vi "NI PXI-4110 Programmable Power Supply Ch Page.vi"(8 "error in (no error)":errorcluster, 11 "Node Ptr":T3 format="%.0x") -> (0 "error out":errorcluster)   [LabVIEW 2015, in "NI PXI-4110 Programmable Power Supply Custom Device.lvlib"]
uses:
  NI PXI-4110 Programmable Power Supply Custom Device.lvlib
  <vilib>/NI Veristand/Custom Device API/Custom Device Item Ref.ctl
  <instrlib>/niDCPower/nidcpower.llb/niDCPower Sense.ctl
  4110_Channel #.ctl
  4110_Global.vi
  <vilib>/NI Veristand/Custom Device API/Get Item Property (U16).vi
  <vilib>/NI Veristand/Custom Device API/Get Item Property (Double).vi
  <vilib>/NI Veristand/Custom Device API/Get Item Property (I32).vi
  <vilib>/NI Veristand/Custom Device API/Set Item Property (I32).vi
  <vilib>/NI Veristand/Custom Device API/Set Item Property (U16).vi
  <vilib>/NI Veristand/Custom Device API/Set Item Property (Double).vi
  <vilib>/NI VeriStand/Custom Device API/Custom Device API.lvlib
panel:
  in  "Channel #":T1
  in  "Voltage Limit":dbl caption="Range (0-6V)" format="%.4f"
  in  "Initial Current Value":dbl caption="Range (0.01 -1A)" format="%.4f"
  in  "Current Limit":dbl caption="Range (0.01-1A)" format="%.4f"
  in  "sense":T2=1008 caption="Sense" items=["Local"=1008, "Remote"=1009]
  in  "IO Type":enum16{"Voltage Output", "Current Output"}(ring)
  in  "Initial Voltage Value":dbl caption="Range (0-6V)" format="%_4f"
  in  "Name":string
  in  "Header":cluster{"Section Name":string}={"Section Name"="PXI-4110  Settings"}
  in  "Description":string
  in  "Delete":bool
  # "Voltage  IO Settings"
  # "Current IO Settings"
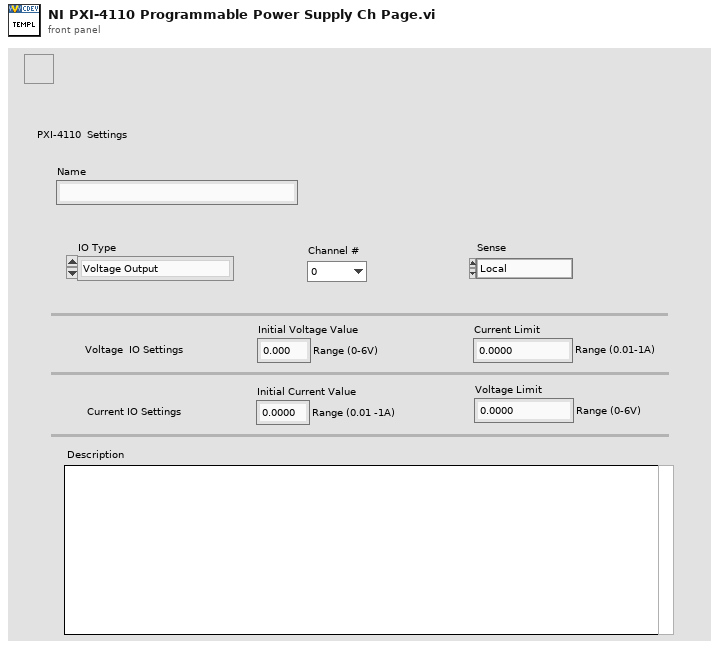
[diagram p1: front panel]
types:
  T1 = typedef "NI PXI-4110 Programmable Power Supply Custom Device.lvlib/4110_Channel #.ctl" = enum16{"0", "1", "2"}
  T2 = typedef "niDCPower Sense.ctl" = i32
  T3 = typedef "Custom Device API.lvlib/Custom Device Item Ref.ctl" = u64
  T4 = enum8{"Enabled", "Disabled", "Disabled and Grayed Out"}
  T5 = typedef "Custom Device API.lvlib/Custom Device Item Info.ctl" = cluster{"Name":string, "Is Channel":bool, "GUID":string, "Is Waveform":bool}
  T6 = cluster{"V_min":dbl, "V_max":dbl, "I_min":dbl, "I_max":dbl}
  T7 = typedef "Custom Device API.lvlib/Custom Device Commands.ctl" = enum16{"Default", "Item renamed", "Shutdown", "Dynamic button pressed"}
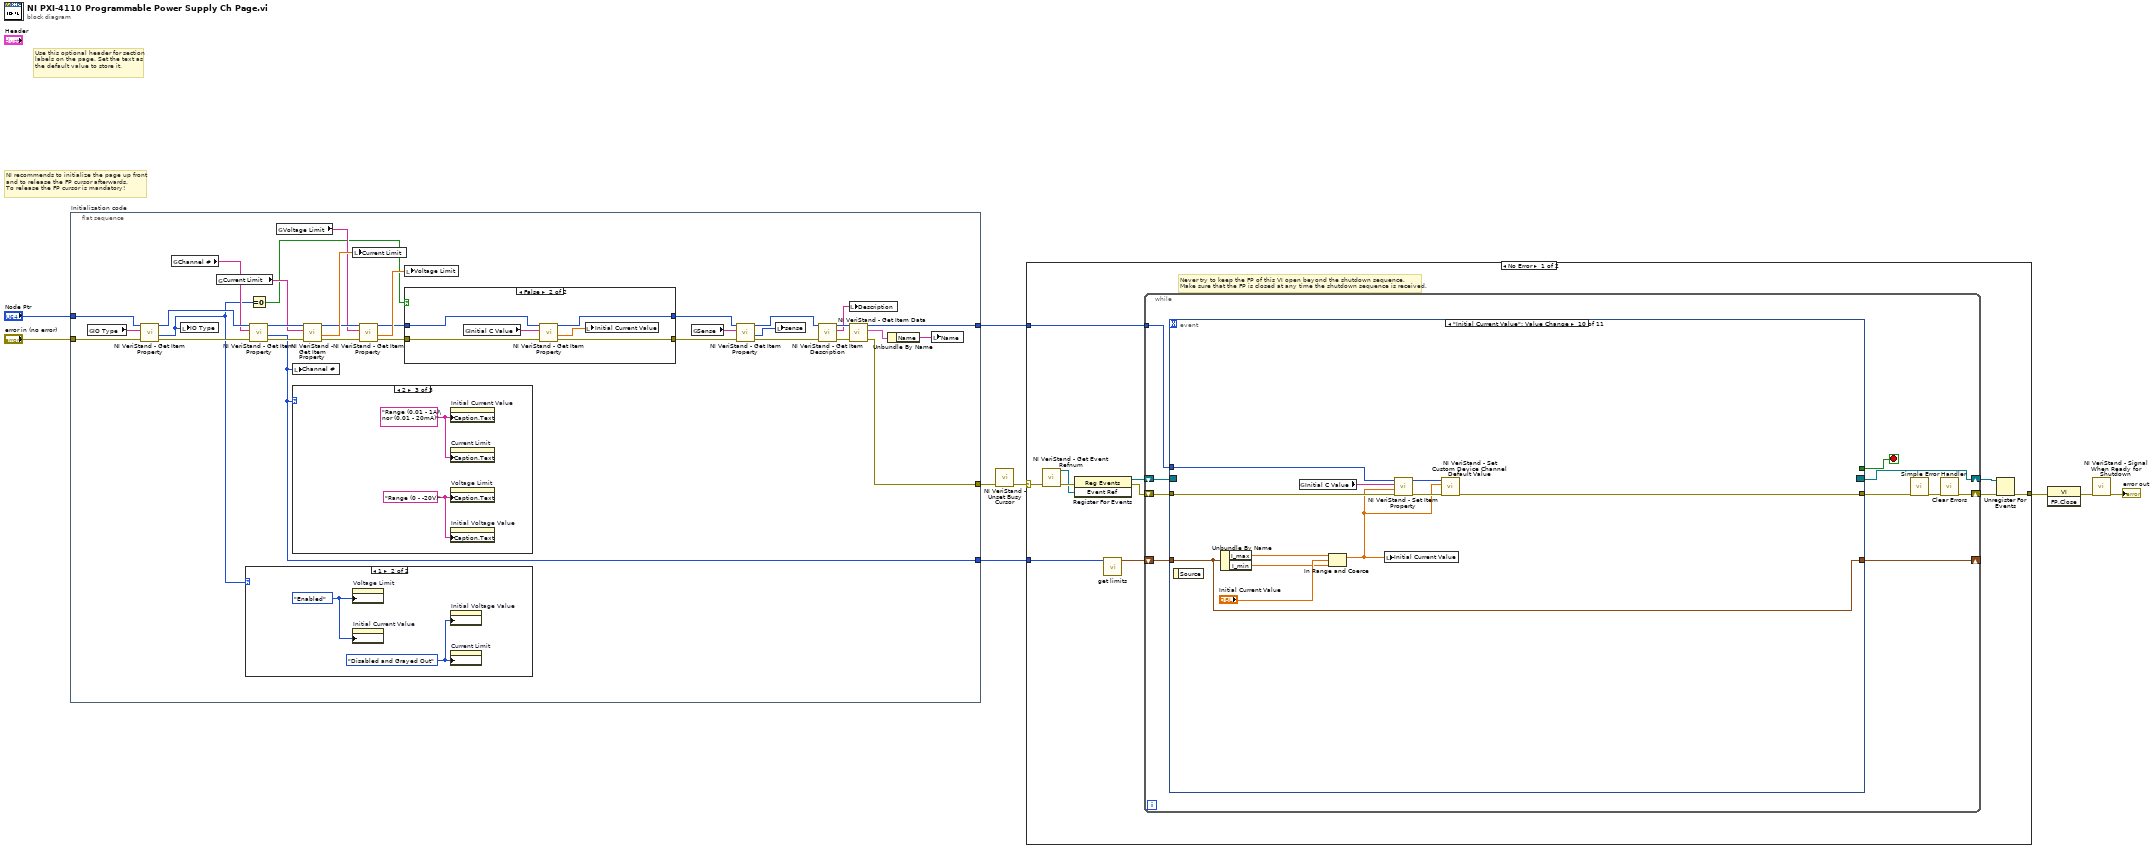
[diagram p0: block diagram]
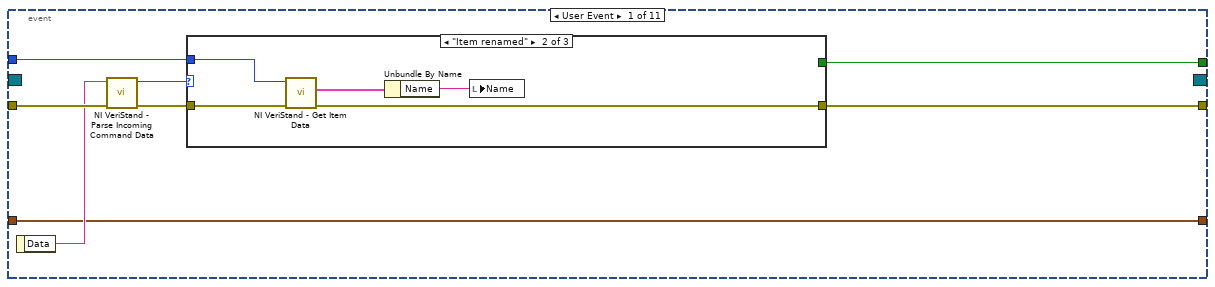
[diagram p2: hidden frame]
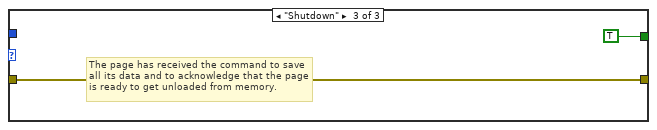
[diagram p4: hidden frame]
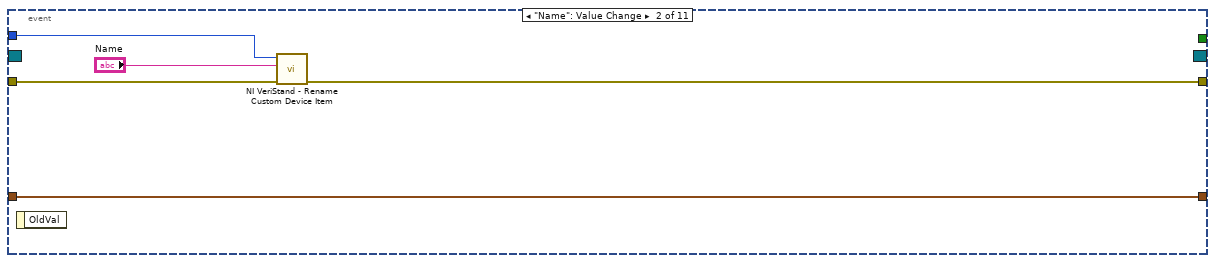
[diagram p5: hidden frame]
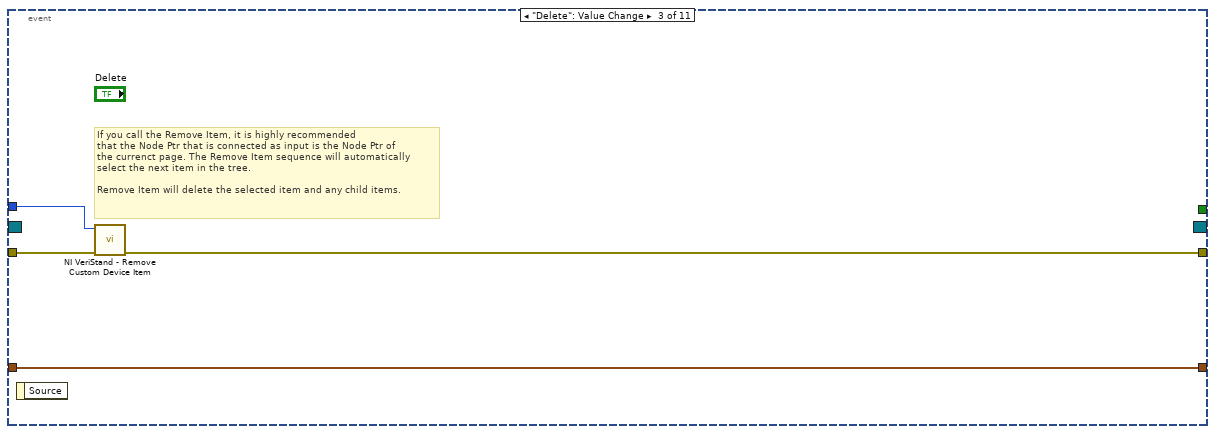
[diagram p6: hidden frame]
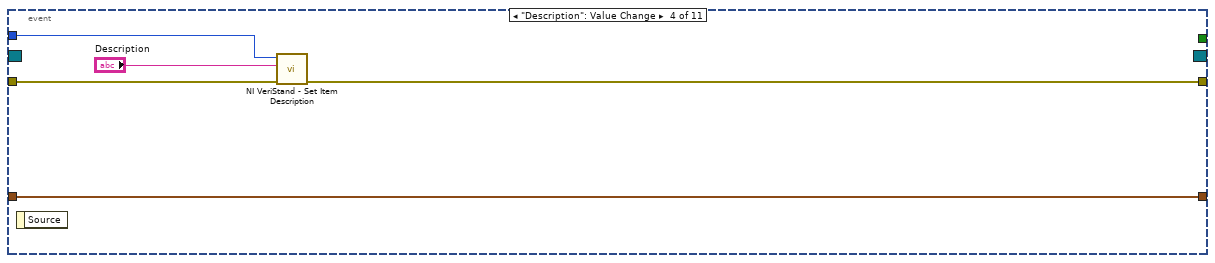
[diagram p7: hidden frame]
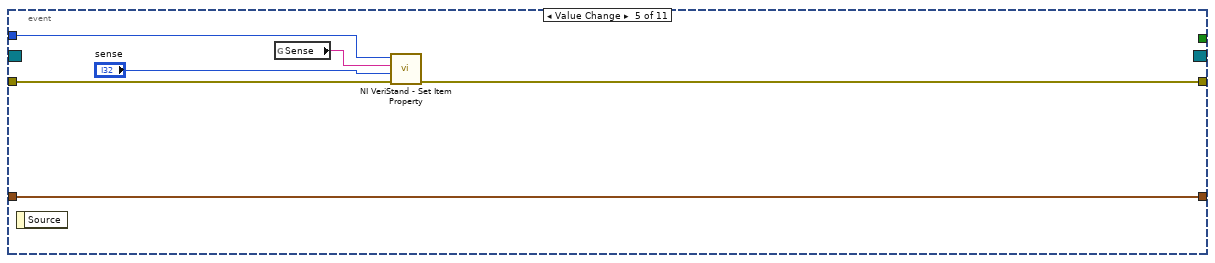
[diagram p8: hidden frame]
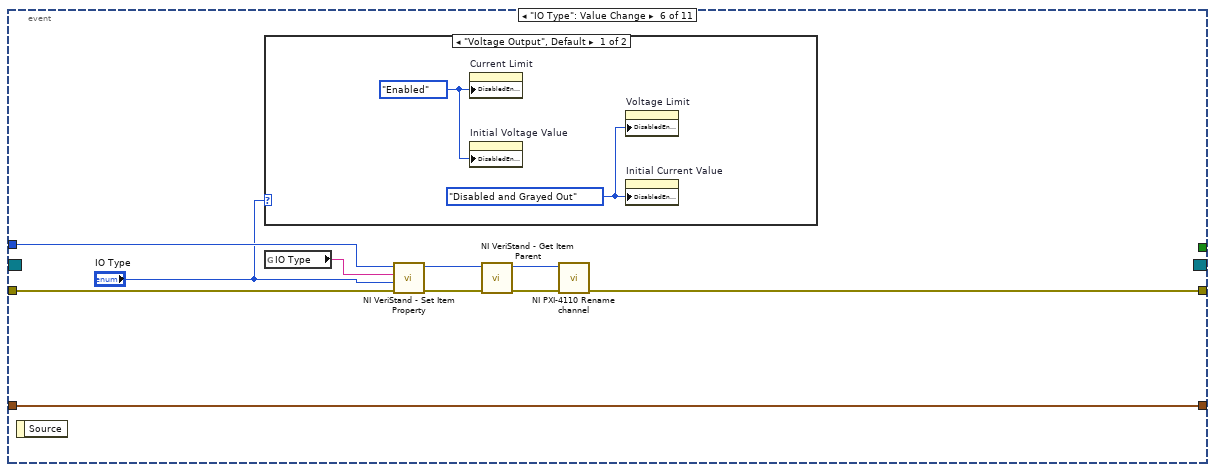
[diagram p9: hidden frame]
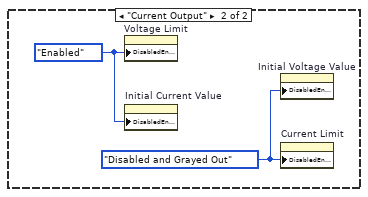
[diagram p10: hidden frame]
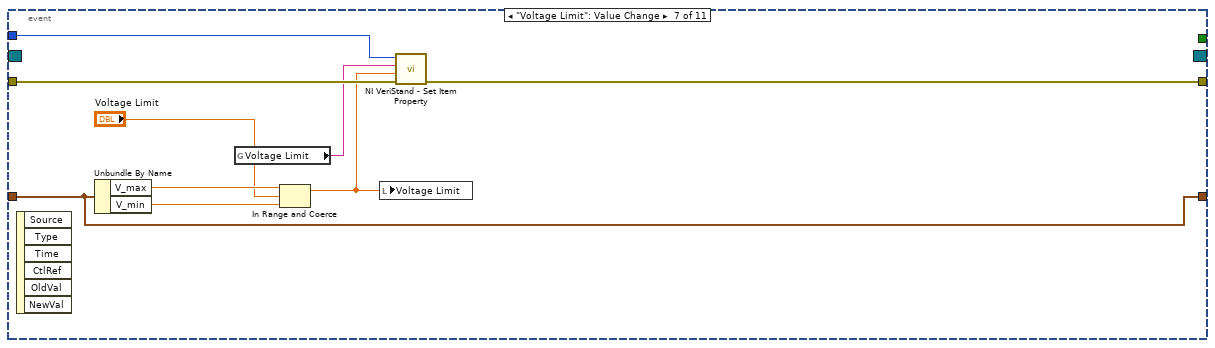
[diagram p11: hidden frame]
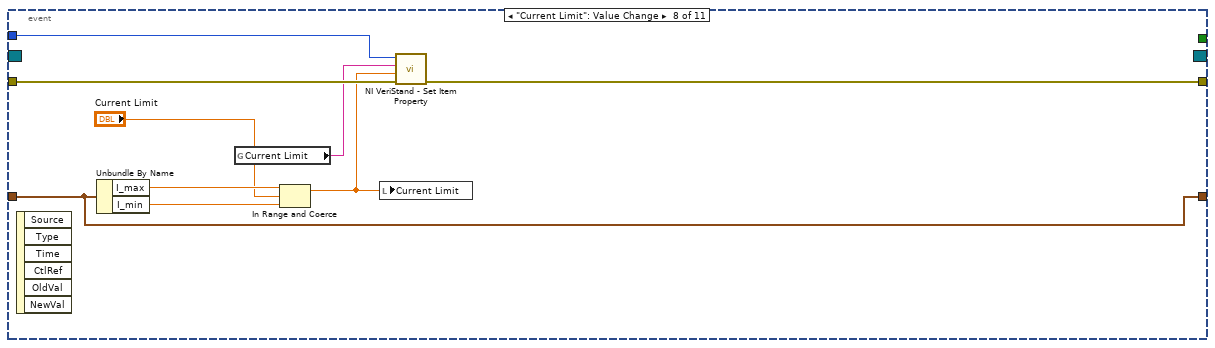
[diagram p12: hidden frame]
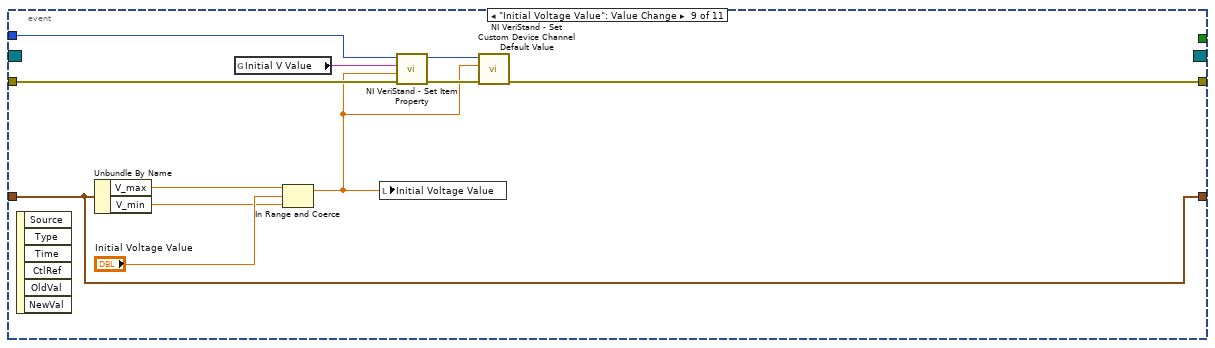
[diagram p13: hidden frame]
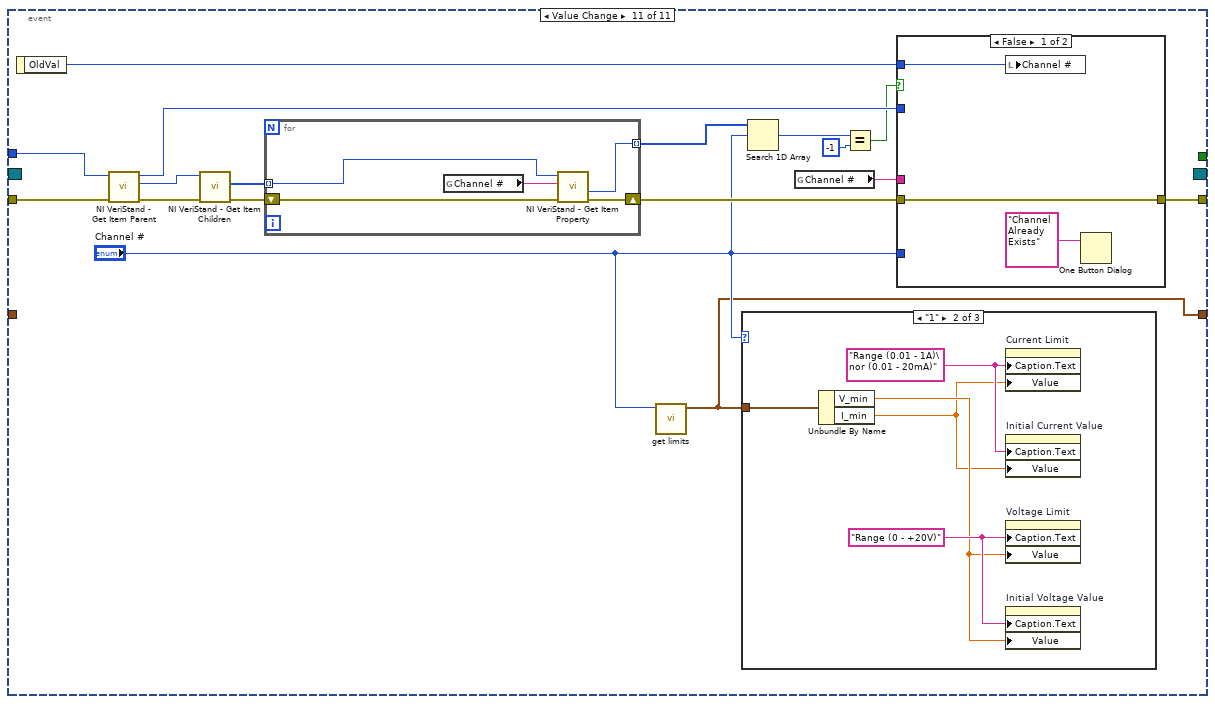
[diagram p14: hidden frame]
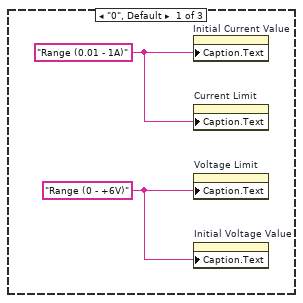
[diagram p15: hidden frame]
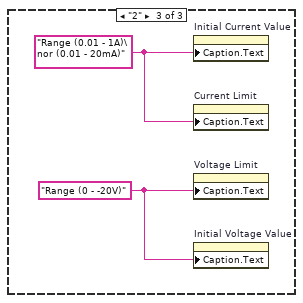
[diagram p16: hidden frame]
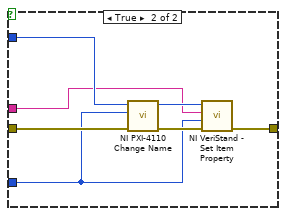
[diagram p17: hidden frame]
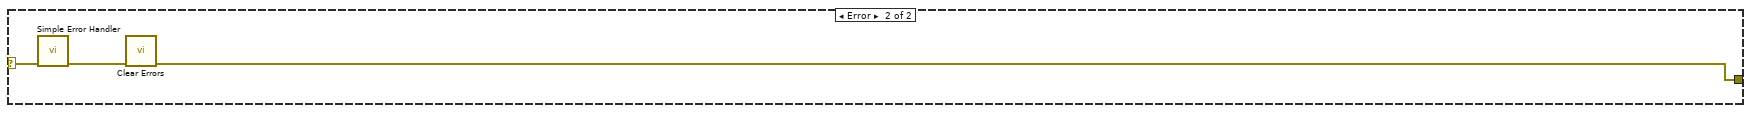
[diagram p18: hidden frame]
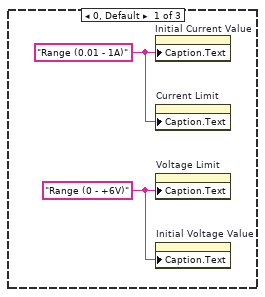
[diagram p19: hidden frame]
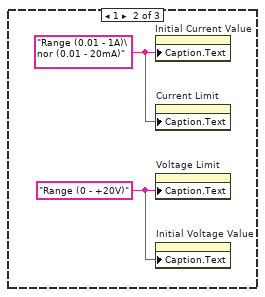
[diagram p20: hidden frame]
diagram:
  # "Use this optional header for section labels on the page. Set the text as the default value to store it."
  # "NI recommends to initialize the page up front\nand to release the FP cursor afterwards.\nTo release the FP cursor is mandatory!"
  n1 = flat-sequence "Initialization code" {
    tunnel: "error in (no error)" -> [w34]
    tunnel: "Node Ptr" -> [w33]
    tunnel: [w36] -> w5
    tunnel: [w41] -> w3
    tunnel: [w10] -> w1
    frame #0 {
      n2 = global read "4110_Global.vi" "IO Type"() -> (w32:string)
      n3 = call-poly <vilib>:"NI VeriStand - Get Item Property.vi"("error in (no error)"=w34, "Property Name"=w32, "Item Ref in"=w33) -> ("error out"=w31:errorcluster, "Value"=w12:u16, "Item Ref out"=w30:T3)  [unwired: 5 in, 1 out]
      n4 = global read "4110_Global.vi" "Channel #"() -> (w29:string)
      n5 = local write "IO Type"(w12) -> ()
      n6 = global read "4110_Global.vi" "Current Limit"() -> (w26:string)
      n7 = case shown="1" w12 {
        frame 0, Default {
          w60 = T4."Enabled" ("Disabled")
          w61 = T4."Disabled and Grayed Out" ("Disabled")
          n8 = property on="Current Limit" class="DigNum (strict)"("DisabledEnum"=w60) -> ()  [unwired: 2 in, 2 out]
          n9 = property on="Initial Voltage Value" class="DigNum (strict)"("DisabledEnum"=w60) -> ()  [unwired: 2 in, 2 out]
          n10 = property on="Voltage Limit" class="DigNum (strict)"("DisabledEnum"=w61) -> ()  [unwired: 2 in, 2 out]
          n11 = property on="Initial Current Value" class="DigNum (strict)"("DisabledEnum"=w61) -> ()  [unwired: 2 in, 2 out]
        }
        frame 1 {
          w62 = T4."Enabled" ("Disabled")
          w63 = T4."Disabled and Grayed Out" ("Disabled")
          n12 = property on="Voltage Limit" class="DigNum (strict)"("DisabledEnum"=w62) -> ()  [unwired: 2 in, 2 out]
          n13 = property on="Initial Current Value" class="DigNum (strict)"("DisabledEnum"=w62) -> ()  [unwired: 2 in, 2 out]
          n14 = property on="Initial Voltage Value" class="DigNum (strict)"("DisabledEnum"=w63) -> ()  [unwired: 2 in, 2 out]
          n15 = property on="Current Limit" class="DigNum (strict)"("DisabledEnum"=w63) -> ()  [unwired: 2 in, 2 out]
        }
      }
      n16 = Equal To 0?(x=w12) -> (x = 0?=w11:bool)
      n17 = call-poly <vilib>:"NI VeriStand - Get Item Property.vi"("error in (no error)"=w31, "Property Name"=w29, "Item Ref in"=w30) -> ("error out"=w27:errorcluster, "Value"=w10:u16, "Item Ref out"=w28:T3)  [unwired: 5 in, 1 out]
      n18 = global read "4110_Global.vi" "Voltage Limit"() -> (w22:string)
      n19 = local write "Channel #"(w10) -> ()
      n20 = case shown="2" w10 {
        frame 0, Default {
          w42 = "Range (0 - +6V)" ("Caption.Text")
          w43 = "Range (0.01 - 1A)" ("Caption.Text")
          n21 = property on="Initial Current Value" class="DigNum (strict)"("Caption.Text"=w43) -> ()  [unwired: 2 in, 2 out]
          n22 = property on="Current Limit" class="DigNum (strict)"("Caption.Text"=w43) -> ()  [unwired: 2 in, 2 out]
          n23 = property on="Voltage Limit" class="DigNum (strict)"("Caption.Text"=w42) -> ()  [unwired: 2 in, 2 out]
          n24 = property on="Initial Voltage Value" class="DigNum (strict)"("Caption.Text"=w42) -> ()  [unwired: 2 in, 2 out]
        }
        frame 1 {
          w44 = "Range (0 - +20V)" ("Caption.Text")
          w45 = "Range (0.01 - 1A)\nor (0.01 - 20mA)" ("Caption.Text")
          n25 = property on="Initial Current Value" class="DigNum (strict)"("Caption.Text"=w45) -> ()  [unwired: 2 in, 2 out]
          n26 = property on="Current Limit" class="DigNum (strict)"("Caption.Text"=w45) -> ()  [unwired: 2 in, 2 out]
          n27 = property on="Voltage Limit" class="DigNum (strict)"("Caption.Text"=w44) -> ()  [unwired: 2 in, 2 out]
          n28 = property on="Initial Voltage Value" class="DigNum (strict)"("Caption.Text"=w44) -> ()  [unwired: 2 in, 2 out]
        }
        frame 2 {
          w46 = "Range (0 - -20V)" ("Caption.Text")
          w47 = "Range (0.01 - 1A)\nor (0.01 - 20mA)" ("Caption.Text")
          n29 = property on="Initial Current Value" class="DigNum (strict)"("Caption.Text"=w47) -> ()  [unwired: 2 in, 2 out]
          n30 = property on="Current Limit" class="DigNum (strict)"("Caption.Text"=w47) -> ()  [unwired: 2 in, 2 out]
          n31 = property on="Voltage Limit" class="DigNum (strict)"("Caption.Text"=w46) -> ()  [unwired: 2 in, 2 out]
          n32 = property on="Initial Voltage Value" class="DigNum (strict)"("Caption.Text"=w46) -> ()  [unwired: 2 in, 2 out]
        }
      }
      n33 = call-poly <vilib>:"NI VeriStand - Get Item Property.vi"("error in (no error)"=w27, "Property Name"=w26, "Item Ref in"=w28) -> ("error out"=w24:errorcluster, "Value"=w25:dbl, "Item Ref out"=w23:T3)  [unwired: 5 in, 1 out]
      n34 = local write "Current Limit"(w25) -> ()
      n35 = call-poly <vilib>:"NI VeriStand - Get Item Property.vi"("error in (no error)"=w24, "Property Name"=w22, "Item Ref in"=w23) -> ("error out"=w19:errorcluster, "Value"=w21:dbl, "Item Ref out"=w20:T3)  [unwired: 5 in, 1 out]
      n36 = local write "Voltage Limit"(w21) -> ()
      n37 = case shown="False" w11 {
        tunnel: w20 -> [w53 w59]
        tunnel: w19 -> [w52 w58]
        tunnel: [w51 w57] -> w17
        tunnel: [w50 w56] -> w16
        frame True {
          n38 = global read "4110_Global.vi" "Initial V Value"() -> (w49:string)
          n39 = call-poly <vilib>:"NI VeriStand - Get Item Property.vi"("error in (no error)"=w52, "Property Name"=w49, "Item Ref in"=w53) -> ("error out"=w51:errorcluster, "Value"=w48:dbl, "Item Ref out"=w50:T3)  [unwired: 5 in, 1 out]
          n40 = local write "Initial Voltage Value"(w48) -> ()
        }
        frame False {
          n41 = global read "4110_Global.vi" "Initial C Value"() -> (w55:string)
          n42 = call-poly <vilib>:"NI VeriStand - Get Item Property.vi"("error in (no error)"=w58, "Property Name"=w55, "Item Ref in"=w59) -> ("error out"=w57:errorcluster, "Value"=w54:dbl, "Item Ref out"=w56:T3)  [unwired: 5 in, 1 out]
          n43 = local write "Initial Current Value"(w54) -> ()
        }
      }
      n44 = global read "4110_Global.vi" "Sense"() -> (w15:string)
      n45 = call-poly <vilib>:"NI VeriStand - Get Item Property.vi"("error in (no error)"=w17, "Property Name"=w15, "Item Ref in"=w16) -> ("error out"=w13:errorcluster, "Value"=w18:i32, "Item Ref out"=w14:T3)  [unwired: 5 in, 1 out]
      n46 = local write "sense"(w18) -> ()
      n47 = call <vilib>:"NI VeriStand - Get Item Description.vi"("error in (no error)"=w13, "Item Ref in"=w14) -> ("error out"=w38:errorcluster, "Description"=w39:string, "Item Ref out"=w40:T3)  [unwired: 7 out]
      n48 = local write "Description"(w39) -> ()
      n49 = call <vilib>:"NI VeriStand - Get Item Data.vi"("error in (no error)"=w38, "Item Ref in"=w40) -> ("error out"=w36:errorcluster, "Item Info"=w37:T5, "Item Ref out"=w41:T3)  [unwired: 7 out]
      n50 = Unbundle By Name(w37) -> ("Name"=w35:string)
      n51 = local write "Name"(w35) -> ()
    }
  }
  n52 = call <vilib>:"NI VeriStand - Unset Busy Cursor.vi"("error in (no error)"=w5) -> ("error out"=w4:errorcluster)  [unwired: 10 out]
  n53 = case shown="No Error" w4 {
    selector: w4 -> [w66 w218]
    tunnel: [w71 w216] -> w9
    tunnel: w3 -> [w67 _]
    tunnel: w1 -> [w65 _]
    frame No Error {
      # "Never try to keep the FP of this VI open beyond the shutdown sequence.\nMake sure that the FP is closed at any time the shutdown sequence is received."
      n54 = call <vilib>:"NI VeriStand - Get Event Refnum.vi"("error in (no error)"=w66) -> ("error out"=w74:errorcluster, "Event Ref"=w70:refnum<user-event>)  [unwired: 9 out]
      n55 = register-events(error in=w74, w70) -> (reference out=w68:refnum<event-registration>, error out=w69:errorcluster)  [unwired: 1 in]
      n56 = call "get limits.vi"("Channel #"=w65) -> ("output cluster"=w64:T6)  [unwired: 10 in]
      n57 = while {
        tunnel: w67 -> [w80]
        shift-right: [w77] -> w72
        shift-left: w69 -> [w83]
        shift-right: [w84] -> w73
        shift-left: w68 -> [w82]
        shift-right: [w76] -> _
        shift-left: w64 -> [w75]
        stop <- w81 stop-if-true
        n58 = event shown="[9] \"Initial Current Value\": Value Change" {
          selector: w82 -> [_ _ _ _ _ _ _ _ _ _ _]
          dyn-events: [_ _ _ _ _ _ _ _ _ _ _] -> w84
          timeout: _ -> [_ _ _ _ _ _ _ _ _ _ _]
          tunnel: w83 -> [w92 w105 w109 w113 w120 w129 w142 w151 w162 w173 w178]
          tunnel: [w88 _ _ _ _ _ _ _ _ _ _] -> w81
          tunnel: [w87 w104 w108 w112 w119 w123 w141 w150 w159 w171 w177] -> w79
          tunnel: w80 -> [w86 w103 w107 w114 w118 w130 w143 w152 w163 w174 w179]
          tunnel: [w85 w101 w106 w110 w115 w121 w139 w147 w155 w168 w175] -> w76
          tunnel: w75 -> [w85 w101 w106 w110 w115 w121 w139 w147 w155 w168 _]
          event User Event {
            n59 = event-data() -> ("Data"=w91:string)  [unwired: 1 out]
            n60 = call <vilib>:"NI VeriStand - Parse Incoming Command Data.vi"("error in (no error)"=w92, "Incoming data"=w91) -> ("error out"=w90:errorcluster, "Action"=w89:T7)  [unwired: 8 out]
            n61 = case shown="\"Item renamed\"" w89 {
              tunnel: w90 -> [w93 w98 w99]
              tunnel: [_ _ TRUE] -> w88
              tunnel: [w93 w95 w99] -> w87
              tunnel: w86 -> [_ w97 _]
              frame "Default", Default {
              }
              frame "Item renamed" {
                n62 = call <vilib>:"NI VeriStand - Get Item Data.vi"("error in (no error)"=w98, "Item Ref in"=w97) -> ("error out"=w95:errorcluster, "Item Info"=w96:T5)  [unwired: 8 out]
                n63 = Unbundle By Name(w96) -> ("Name"=w94:string)
                n64 = local write "Name"(w94) -> ()
              }
              frame "Shutdown" {
                # "The page has received the command to save all its data and to acknowledge that the page is ready to get unloaded from memory."
              }
            }
          }
          event "Name": Value Change {
            n65 = event-data() -> ()  [unwired: 2 out]
            n66 = call <vilib>:"NI VeriStand - Rename Custom Device Item.vi"("error in (no error)"=w105, "New Name"="Name", "Item Ref in"=w103) -> ("error out"=w104:errorcluster)  [unwired: 1 in, 7 out]
          }
          event "Delete": Value Change {
            # "If you call the Remove Item, it is highly recommended\nthat the Node Ptr that is connected as input is the Node Ptr of\nthe currenct page. The Remove Item sequence will automatically\nselect the next item in the tree.\n\nRemove Item will delete the selected item and any child items."
            n67 = event-data() -> ()  [unwired: 2 out]
            n68 = call <vilib>:"NI VeriStand - Remove Custom Device Item.vi"("error in (no error)"=w109, "Item Ref in"=w107) -> ("error out"=w108:errorcluster)  [unwired: 1 in, 8 out]
          }
          event "Description": Value Change {
            n69 = event-data() -> ()  [unwired: 2 out]
            n70 = call <vilib>:"NI VeriStand - Set Item Description.vi"("error in (no error)"=w113, "Description"="Description", "Item Ref in"=w114) -> ("error out"=w112:errorcluster)  [unwired: 8 out]
          }
          event Value Change {
            n71 = event-data() -> ()  [unwired: 2 out]
            n72 = global read "4110_Global.vi" "Sense"() -> (w117:string)
            n73 = call-poly <vilib>:"NI VeriStand - Set Item Property.vi"("error in (no error)"=w120, "Value"="sense", "Property Name"=w117, "Item Ref in"=w118) -> ("error out"=w119:errorcluster)  [unwired: 5 in, 2 out]
          }
          event "IO Type": Value Change {
            n74 = event-data() -> ()  [unwired: 2 out]
            n75 = case shown="\"Voltage Output\", Default" "IO Type" {
              frame "Voltage Output", Default {
                w131 = T4."Enabled" ("Disabled")
                w132 = T4."Disabled and Grayed Out" ("Disabled")
                n76 = property on="Current Limit" class="DigNum (strict)"("DisabledEnum"=w131) -> ()  [unwired: 2 in, 2 out]
                n77 = property on="Initial Voltage Value" class="DigNum (strict)"("DisabledEnum"=w131) -> ()  [unwired: 2 in, 2 out]
                n78 = property on="Voltage Limit" class="DigNum (strict)"("DisabledEnum"=w132) -> ()  [unwired: 2 in, 2 out]
                n79 = property on="Initial Current Value" class="DigNum (strict)"("DisabledEnum"=w132) -> ()  [unwired: 2 in, 2 out]
              }
              frame "Current Output" {
                w133 = T4."Enabled" ("Disabled")
                w134 = T4."Disabled and Grayed Out" ("Disabled")
                n80 = property on="Voltage Limit" class="DigNum (strict)"("DisabledEnum"=w133) -> ()  [unwired: 2 in, 2 out]
                n81 = property on="Initial Current Value" class="DigNum (strict)"("DisabledEnum"=w133) -> ()  [unwired: 2 in, 2 out]
                n82 = property on="Initial Voltage Value" class="DigNum (strict)"("DisabledEnum"=w134) -> ()  [unwired: 2 in, 2 out]
                n83 = property on="Current Limit" class="DigNum (strict)"("DisabledEnum"=w134) -> ()  [unwired: 2 in, 2 out]
              }
            }
            n84 = global read "4110_Global.vi" "IO Type"() -> (w128:string)
            n85 = call-poly <vilib>:"NI VeriStand - Set Item Property.vi"("error in (no error)"=w129, "Value"="IO Type", "Property Name"=w128, "Item Ref in"=w130) -> ("error out"=w126:errorcluster, "Item Ref out"=w124:T3)  [unwired: 5 in, 1 out]
            n86 = call <vilib>:"NI VeriStand - Get Item Parent.vi"("error in (no error)"=w126, "Item Ref in"=w124) -> ("error out"=w122:errorcluster, "Item Ref out"=w125:T3)  [unwired: 6 in, 2 out]
            n87 = call "NI PXI-4110 Rename channel.vi"("error in (no error)"=w122, "Node Ptr"=w125) -> ("error out"=w123:errorcluster)  [unwired: 8 in, 1 out]
          }
          event "Voltage Limit": Value Change {
            n88 = event-data() -> ()  [unwired: 7 out]
            n89 = Unbundle By Name(w139) -> ("V_max"=w138:dbl, "V_min"=w137:dbl)
            n90 = global read "4110_Global.vi" "Voltage Limit"() -> (w140:string)
            n91 = In Range and Coerce(upper limit=w138, x="Voltage Limit", lower limit=w137) -> (coerced(x)=w135:dbl)  [unwired: 1 out]
            n92 = local write "Voltage Limit"(w135) -> ()
            n93 = call-poly <vilib>:"NI VeriStand - Set Item Property.vi"("error in (no error)"=w142, "Value"=w135, "Property Name"=w140, "Item Ref in"=w143) -> ("error out"=w141:errorcluster)  [unwired: 5 in, 2 out]
          }
          event "Current Limit": Value Change {
            n94 = event-data() -> ()  [unwired: 7 out]
            n95 = Unbundle By Name(w147) -> ("I_max"=w149:dbl, "I_min"=w148:dbl)
            n96 = global read "4110_Global.vi" "Current Limit"() -> (w144:string)
            n97 = In Range and Coerce(upper limit=w149, x="Current Limit", lower limit=w148) -> (coerced(x)=w145:dbl)  [unwired: 1 out]
            n98 = local write "Current Limit"(w145) -> ()
            n99 = call-poly <vilib>:"NI VeriStand - Set Item Property.vi"("error in (no error)"=w151, "Value"=w145, "Property Name"=w144, "Item Ref in"=w152) -> ("error out"=w150:errorcluster)  [unwired: 5 in, 2 out]
          }
          event "Initial Voltage Value": Value Change {
            n100 = event-data() -> ()  [unwired: 7 out]
            n101 = Unbundle By Name(w155) -> ("V_max"=w154:dbl, "V_min"=w153:dbl)
            n102 = global read "4110_Global.vi" "Initial V Value"() -> (w161:string)
            n103 = In Range and Coerce(upper limit=w154, x="Initial Voltage Value", lower limit=w153) -> (coerced(x)=w158:dbl)  [unwired: 1 out]
            n104 = local write "Initial Voltage Value"(w158) -> ()
            n105 = call-poly <vilib>:"NI VeriStand - Set Item Property.vi"("error in (no error)"=w162, "Value"=w158, "Property Name"=w161, "Item Ref in"=w163) -> ("error out"=w160:errorcluster, "Item Ref out"=w157:T3)  [unwired: 5 in, 1 out]
            n106 = call <vilib>:"NI VeriStand - Set Custom Device Channel Default Value.vi"("error in (no error)"=w160, "Default Value"=w158, "Channel Ref in"=w157) -> ("error out"=w159:errorcluster)  [unwired: 7 in, 1 out]
          }
          event "Initial Current Value": Value Change {
            n107 = event-data() -> ()  [unwired: 2 out]
            n108 = Unbundle By Name(w168) -> ("I_max"=w167:dbl, "I_min"=w166:dbl)
            n109 = global read "4110_Global.vi" "Initial C Value"() -> (w164:string)
            n110 = In Range and Coerce(upper limit=w167, x="Initial Current Value", lower limit=w166) -> (coerced(x)=w165:dbl)  [unwired: 1 out]
            n111 = local write "Initial Current Value"(w165) -> ()
            n112 = call-poly <vilib>:"NI VeriStand - Set Item Property.vi"("error in (no error)"=w173, "Value"=w165, "Property Name"=w164, "Item Ref in"=w174) -> ("error out"=w172:errorcluster, "Item Ref out"=w170:T3)  [unwired: 5 in, 1 out]
            n113 = call <vilib>:"NI VeriStand - Set Custom Device Channel Default Value.vi"("error in (no error)"=w172, "Default Value"=w165, "Channel Ref in"=w170) -> ("error out"=w171:errorcluster)  [unwired: 7 in, 1 out]
          }
          event Value Change {
            n114 = event-data() -> ("OldVal"=w181:T1)  [unwired: 1 out]
            n115 = call <vilib>:"NI VeriStand - Get Item Parent.vi"("error in (no error)"=w178, "Item Ref in"=w179) -> ("error out"=w182:errorcluster, "Parent Ref"=w183:T3, "Item Ref out"=w191:T3)  [unwired: 6 in, 1 out]
            n116 = call <vilib>:"NI VeriStand - Get Item Children.vi"("error in (no error)"=w182, "Item Ref in"=w183) -> ("error out"=w185:errorcluster, "Child Refs"=w184:T3[])  [unwired: 6 in, 2 out]
            n117 = for {
              tunnel: w184 -> [w213] mode=indexing
              shift-right: [w214] -> w190
              shift-left: w185 -> [w215]
              tunnel: [w212] -> w186 mode=indexing
              n118 = global read "4110_Global.vi" "Channel #"() -> (w211:string)
              n119 = call-poly <vilib>:"NI VeriStand - Get Item Property.vi"("error in (no error)"=w215, "Property Name"=w211, "Item Ref in"=w213) -> ("error out"=w214:errorcluster, "Value"=w212:u16)  [unwired: 5 in, 2 out]
            }
            n120 = call "get limits.vi"("Channel #"="Channel #") -> ("output cluster"=w175:T6)  [unwired: 10 in]
            n121 = case shown="\"1\"" "Channel #" {
              tunnel: w175 -> [_ w196 _]
              frame "0", Default {
                w192 = "Range (0 - +6V)" ("Caption.Text")
                w193 = "Range (0.01 - 1A)" ("Caption.Text")
                n122 = property on="Initial Current Value" class="DigNum (strict)"("Caption.Text"=w193) -> ()  [unwired: 2 in, 2 out]
                n123 = property on="Current Limit" class="DigNum (strict)"("Caption.Text"=w193) -> ()  [unwired: 2 in, 2 out]
                n124 = property on="Voltage Limit" class="DigNum (strict)"("Caption.Text"=w192) -> ()  [unwired: 2 in, 2 out]
                n125 = property on="Initial Voltage Value" class="DigNum (strict)"("Caption.Text"=w192) -> ()  [unwired: 2 in, 2 out]
              }
              frame "1" {
                w197 = "Range (0 - +20V)" ("Caption.Text")
                w198 = "Range (0.01 - 1A)\nor (0.01 - 20mA)" ("Caption.Text")
                n126 = Unbundle By Name(w196) -> ("V_min"=w195:dbl, "I_min"=w194:dbl)
                n127 = property on="Current Limit" class="DigNum (strict)"("Caption.Text"=w198, "Value"=w194) -> ()  [unwired: 2 in, 2 out]
                n128 = property on="Initial Current Value" class="DigNum (strict)"("Caption.Text"=w198, "Value"=w194) -> ()  [unwired: 2 in, 2 out]
                n129 = property on="Voltage Limit" class="DigNum (strict)"("Caption.Text"=w197, "Value"=w195) -> ()  [unwired: 2 in, 2 out]
                n130 = property on="Initial Voltage Value" class="DigNum (strict)"("Caption.Text"=w197, "Value"=w195) -> ()  [unwired: 2 in, 2 out]
              }
              frame "2" {
                w199 = "Range (0 - -20V)" ("Caption.Text")
                w200 = "Range (0.01 - 1A)\nor (0.01 - 20mA)" ("Caption.Text")
                n131 = property on="Initial Current Value" class="DigNum (strict)"("Caption.Text"=w200) -> ()  [unwired: 2 in, 2 out]
                n132 = property on="Current Limit" class="DigNum (strict)"("Caption.Text"=w200) -> ()  [unwired: 2 in, 2 out]
                n133 = property on="Voltage Limit" class="DigNum (strict)"("Caption.Text"=w199) -> ()  [unwired: 2 in, 2 out]
                n134 = property on="Initial Voltage Value" class="DigNum (strict)"("Caption.Text"=w199) -> ()  [unwired: 2 in, 2 out]
              }
            }
            n135 = Search 1D Array(1D array=w186, element="Channel #") -> (index of element=w187:i32)  [unwired: 1 in]
            n136 = global read "4110_Global.vi" "Channel #"() -> (w180:string)
            n137 = Equal?(x=w187, y=-1) -> (x = y?=w189:bool)
            n138 = case shown="False" w189 {
              tunnel: w190 -> [w202 w210]
              tunnel: w191 -> [_ w209]
              tunnel: w180 -> [_ w205]
              tunnel: "Channel #" -> [_ w204]
              tunnel: [w202 w207] -> w177
              tunnel: w181 -> [w203 _]
              frame False {
                n139 = local write "Channel #"(w203) -> ()
                n140 = One Button Dialog(message="Channel Already Exists") -> ()  [unwired: 1 in, 1 out]
              }
              frame True {
                n141 = call "NI PXI-4110 Change Name.vi"("error in (no error)"=w210, "New #"=w204, "Node Ptr"=w209) -> ("error out"=w208:errorcluster, "Node Ptr out"=w206:T3)  [unwired: 7 in]
                n142 = call-poly <vilib>:"NI VeriStand - Set Item Property.vi"("error in (no error)"=w208, "Value"=w204, "Property Name"=w205, "Item Ref in"=w206) -> ("error out"=w207:errorcluster)  [unwired: 5 in, 2 out]
              }
            }
          }
        }
        n143 = call <vilib>:"Simple Error Handler.vi"("error in (no error)"=w79) -> ("error out"=w78:errorcluster)  [unwired: 1 in, 7 out]
        n144 = call <vilib>:"Clear Errors.vi"("error in (no error)"=w78) -> ("error out"=w77:errorcluster)  [unwired: 1 in, 5 out]
      }
      n145 = Unregister For Events(event registration refnum=w73, error in=w72) -> (error out=w71:errorcluster)
    }
    frame Error {
      n146 = call <vilib>:"Simple Error Handler.vi"("error in (no error)"=w218) -> ("error out"=w217:errorcluster)  [unwired: 1 in, 7 out]
      n147 = call <vilib>:"Clear Errors.vi"("error in (no error)"=w217) -> ("error out"=w216:errorcluster)  [unwired: 1 in, 5 out]
    }
  }
  n148 = invoke class="VI" method="FP.Close"(error in=w9) -> (error out=w8:errorcluster)  [unwired: 2 in, 2 out]
  n149 = call <vilib>:"NI VeriStand - Signal When Ready for Shutdown.vi"("error in (no error)"=w8) -> ("error out"=→"error out":errorcluster)  [unwired: 10 out]
